vi "PostLab4.vi"() -> ()   [LabVIEW 2021]
panel:
  out "2D Picture":picture
  in  "Display History":bool
  in  "Size of Rectangle":i16
  out "RecvValue8":dbl
  out "RecvValue7":dbl
  out "RecvValue6":dbl
  out "RecvValue5":dbl
  out "RecvValue4":dbl
  out "RecvValue3":dbl
  out "Y":dbl
  out "X":dbl
  in  "SendValue8":dbl
  in  "SendValue7":dbl
  in  "SendValue6":dbl
  in  "SendValue5":dbl
  in  "SendValue4":dbl
  in  "SendValue3":dbl
  in  "SendValue2":dbl
  in  "SendValue1":dbl
  in  "Send Button":bool
  in  "stop":bool
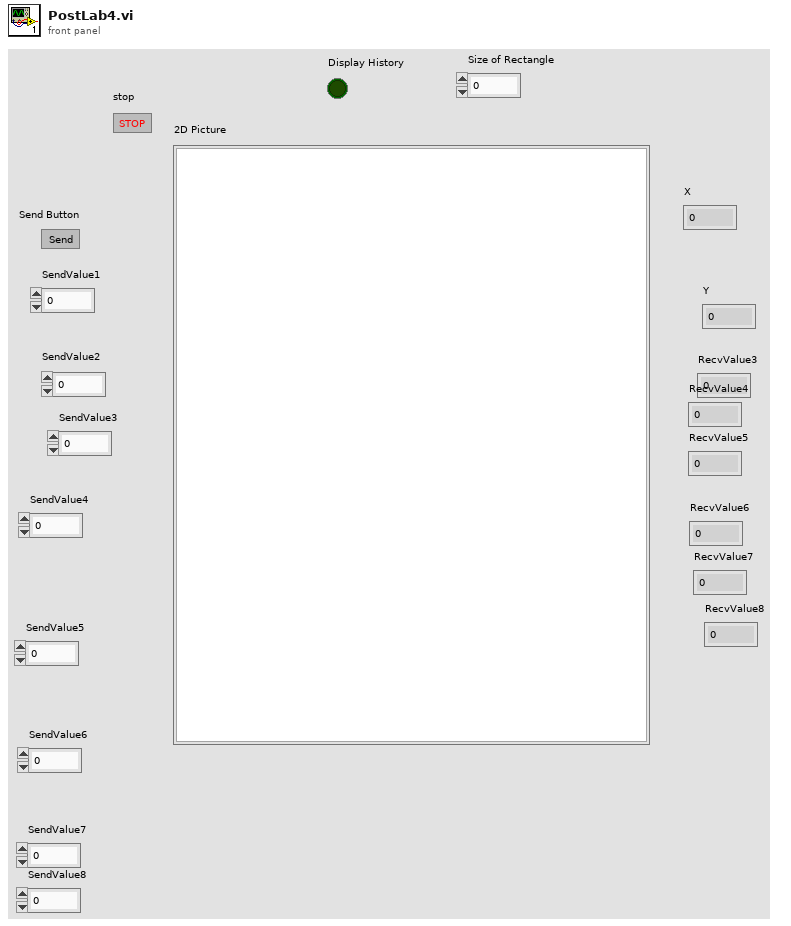
[diagram p1: front panel]
types:
  T1 = enum16{"Standard", "Buffered", "CRLF", "Immediate"}
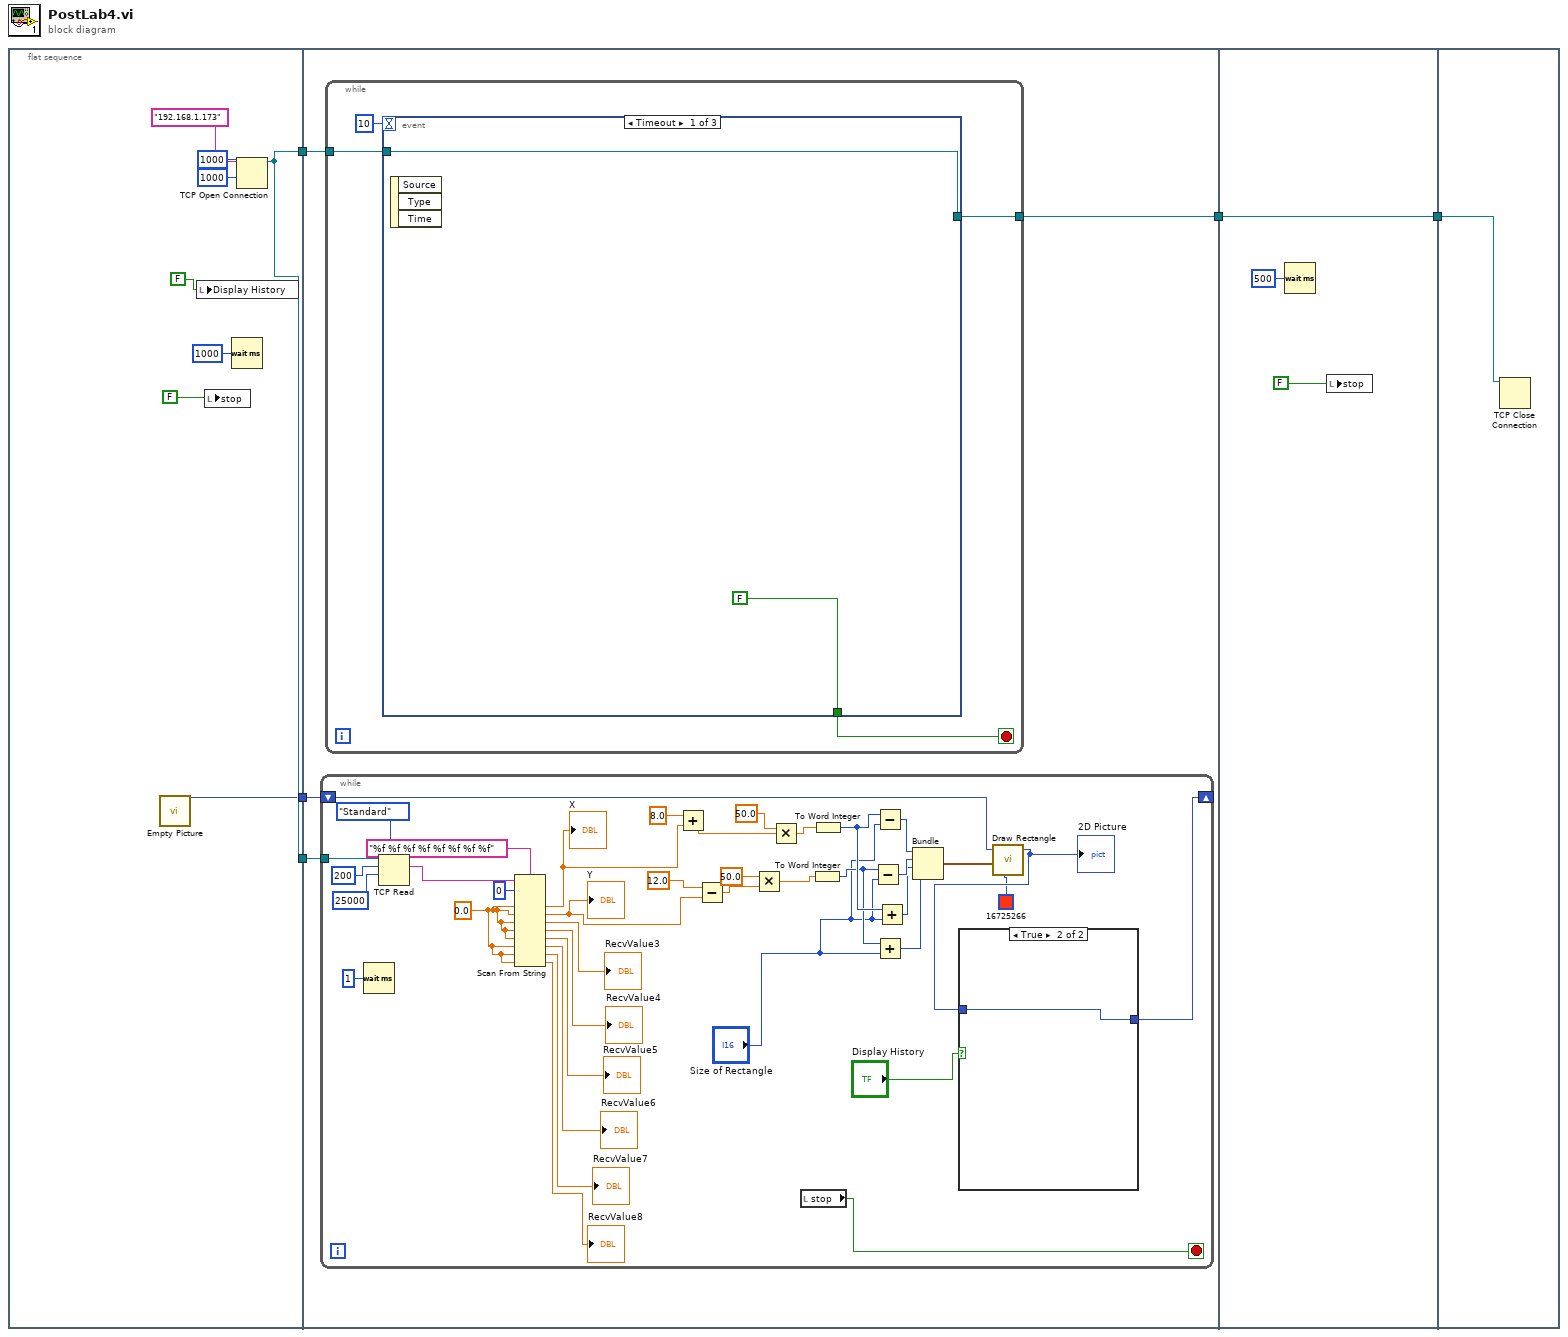
[diagram p0: block diagram]
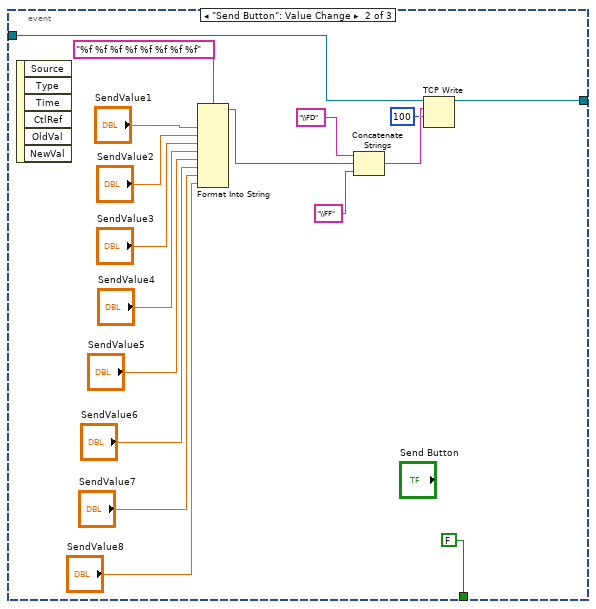
[diagram p3: hidden frame]
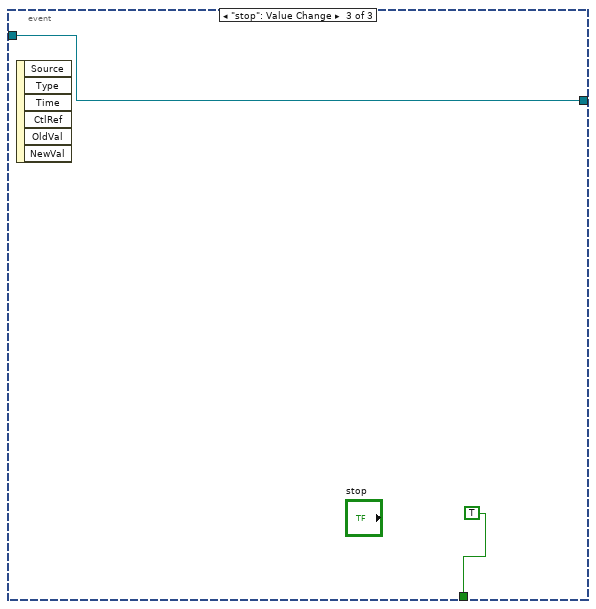
[diagram p4: hidden frame]
diagram:
  n1 = flat-sequence {
    tunnel: [w7] -> w5
    tunnel: [w7] -> w2
    tunnel: [w6] -> w1
    tunnel: w5 -> [w17]
    tunnel: [w16] -> w3
    tunnel: w2 -> [w15]
    tunnel: w1 -> [w14]
    tunnel: [w83] -> w4
    tunnel: w3 -> [w83]
    tunnel: w4 -> [w86]
    frame #0 {
      n2 = call "Empty Picture"() -> ("empty picture"=w6:picture)
      n3 = local write "Display History"(FALSE) -> ()
      n4 = local write "stop"(FALSE) -> ()
      n5 = Wait (ms)(milliseconds to wait=u32 1000) -> ()  [unwired: 1 out]
      n6 = TCP Open Connection(address="192.168.1.173", remote port or service name=u16 1000, timeout ms (60000)=1000) -> (connection ID=w7:refnum<k5>)  [unwired: 2 in, 1 out]
    }
    frame #1 {
      n7 = while {
        tunnel: w15 -> [w55]
        shift-right: [w21] -> _
        shift-left: w14 -> [w23]
        stop <- w18 stop-if-true
        w51 = 0.0 ("default value 1")
        n8 = Wait (ms)(milliseconds to wait=u32 1) -> ()  [unwired: 1 out]
        n9 = TCP Read(connection ID=w55, bytes to read=200, 7:T1."Standard" ("mode (standard)"), 9:25000 ("timeout ms (25000)")) -> (data out=w50:string)  [unwired: 1 in, 2 out]
        n10 = Scan From String(format string="%f %f %f %f %f %f %f %f", input string=w50, initial scan location=u32 0, default 1=w51, default 2=w51, default 3=w51, default 4=w51, default 5=w51, default 6=w51, default 7=w51, default 8=w51) -> (output 1=w41:dbl, output 2=w38:dbl, output 3=→"RecvValue3":dbl, output 4=→"RecvValue4":dbl, output 5=→"RecvValue5":dbl, output 6=→"RecvValue6":dbl, output 7=→"RecvValue7":dbl, output 8=→"RecvValue8":dbl)  [unwired: 1 in, 3 out]
        "X" <- w41
        "Y" <- w38
        n11 = Add(x=8.0, y=w41) -> (x+y=w37:dbl)
        n12 = Subtract(x=12.0, y=w38) -> (x-y=w35:dbl)
        n13 = Multiply(x=50.0, y=w35) -> (x*y=w32:dbl)
        n14 = Multiply(x=50.0, y=w37) -> (x*y=w33:dbl)
        n15 = local read "stop"() -> (w18:bool)
        n16 = To Word Integer(number=w32) -> (16bit integer=w30:i16)
        n17 = To Word Integer(number=w33) -> (16bit integer=w31:i16)
        n18 = Subtract(x=w30, y="Size of Rectangle") -> (x-y=w27:i16)
        n19 = Subtract(x=w31, y="Size of Rectangle") -> (x-y=w28:i16)
        n20 = Add(x=w30, y="Size of Rectangle") -> (x+y=w25:i16)
        n21 = Add(x=w31, y="Size of Rectangle") -> (x+y=w26:i16)
        n22 = Bundle(w28, w27, w26, w25) -> (w20:cluster{i16, i16, i16, i16})  [unwired: 1 in]
        n23 = call <vilib>:"Draw Rectangle.vi"("picture"=w23, "rect"=w20, "color(black)"=u32 16725266) -> ("new picture"=w22:picture)  [unwired: 6 in]
        "2D Picture" <- w22
        n24 = case shown="True" "Display History" {
          tunnel: w22 -> [_ w57]
          tunnel: [_ w57] -> w21
          frame False {
          }
          frame True {
          }
        }
      }
      n25 = while {
        tunnel: w17 -> [w59]
        tunnel: [w58] -> w16
        stop <- w60 stop-if-true
        n26 = event shown="[0] Timeout" {
          selector: _ -> [_ _ _]
          dyn-events: _ -> [_ _ _]
          timeout: 10 -> [_ _ _]
          tunnel: [FALSE FALSE TRUE] -> w60
          tunnel: w59 -> [w62 w65 w81]
          tunnel: [w62 w64 w81] -> w58
          event Timeout {
            n27 = event-data() -> ()  [unwired: 1 in, 3 out]
          }
          event "Send Button": Value Change {
            n28 = event-data() -> ()  [unwired: 1 in, 6 out]
            n29 = Format Into String(format string="%f %f %f %f %f %f %f %f", "SendValue1", "SendValue2", "SendValue3", "SendValue4", "SendValue5", "SendValue6", "SendValue7", "SendValue8") -> (resulting string=w67:string)  [unwired: 2 in, 1 out]
            n30 = Concatenate Strings("\\FD" ("string"), w67, "\\FF" ("string")) -> (w70:string)
            n31 = TCP Write(connection ID=w65, data in=w70, 9:100 ("timeout ms (25000)")) -> (connection ID out=w64:refnum<k5>)  [unwired: 1 in, 2 out]
          }
          event "stop": Value Change {
            n32 = event-data() -> ()  [unwired: 1 in, 6 out]
          }
        }
      }
    }
    frame #2 {
      n33 = Wait (ms)(milliseconds to wait=u32 500) -> ()  [unwired: 1 out]
      n34 = local write "stop"(FALSE) -> ()
    }
    frame #3 {
      n35 = TCP Close Connection(connection ID=w86) -> ()  [unwired: 2 in, 2 out]
    }
  }
